vi "Wing Square Wave Frequency Global.vi"() -> ()   [LabVIEW 2013]
panel:
  in  "Right frequency (periods/tick)":fxp<+,32,0>=0.00390625 caption="frequency (periods/tick)"
  in  "Left frequency (periods/tick)":fxp<+,32,0>=0.00390625 caption="frequency (periods/tick)"
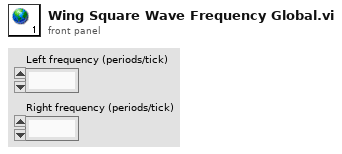
[diagram p1: front panel]
diagram:
